vi "Calc Frame Data .vi"(9 "Rotation Center From Robot Center":T6, 11 "Frame":T5={"Length"=5.0, "Width"=1020.0}) -> (3 "Frame Rotation Set Out":T1 {"Back Right"."Angle" scale format="%.3f"; "Back Right"."Velocity" scale=-1.0..1.0 scale format="%.1f"; "Back Left"."Angle" scale format="%.3f"; "Back Left"."Velocity" scale=-1.0..1.0 scale format="%.1f"; "Front Left"."Angle" scale format="%.3f"; "Front Left"."Velocity" scale=-1.0..1.0 scale format="%.1f"; "Front Right"."Angle" scale format="%.3f"; "Front Right"."Velocity" scale=-1.0..1.0 scale format="%.1f"})   [LabVIEW 2023, in "TShirtWork-SwerveDrive_ACT_ts.lvlib"]
uses:
  TShirtWork-SwerveDrive_ACT_ts.lvlib
  Shared Code/TypeDefs/Cluster_X-Y.ctl
  Type Defs/Cluster_Length and Width.ctl
  Shared Code/TypeDefs/Cluster_Swerve 4 Steer and Velocity.ctl
  Shared Code/TypeDefs/Cluster_Module Velocity-Direction-Rotations.ctl
  Shared Code/TypeDefs/Level_Velocity plus-minus 1.ctl
  Shared Code/TypeDefs/Dial_Compase heading unit circle CCW positive.ctl
  Shared Code/TypeDefs/ENUM_Module Position.ctl
  4e8dd0b3-85a2-4953-8cd2-444eefea6a12.vi
  5d84ef4d-5a06-42ca-b3c1-887b7d6f96c4.vi
panel:
  # "\"Front\" of Robot"
  # "Right Hand Rule"
  # "X"
  # "+CCW"
  # "Y"
  # "(0,0)"
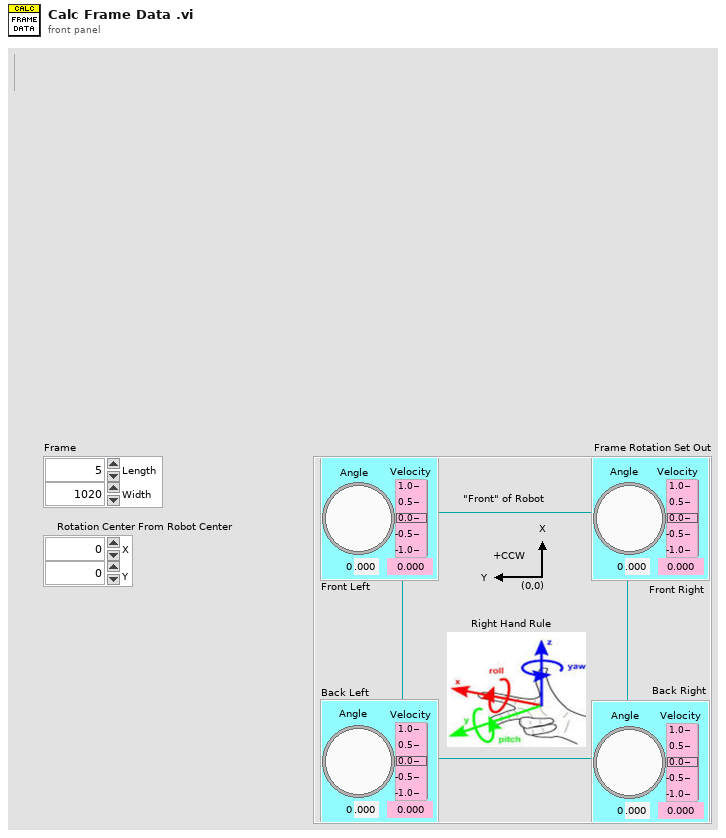
[diagram p1: front panel]
types:
  T1 = typedef "Cluster_Swerve 4 Steer and Velocity.ctl" = cluster{"Front Right":T2, "Front Left":T2, "Back Left":T2, "Back Right":T2}
  T2 = typedef "Cluster_Module Velocity-Direction-Rotations.ctl" = cluster{"Velocity":T3, "Angle":T4, "Rotations Count":dbl}
  T3 = typedef "Level_Velocity plus-minus 1.ctl" = dbl
  T4 = typedef "Dial_Compase heading unit circle CCW positive.ctl" = dbl
  T5 = typedef "Cluster_Length and Width.ctl" = cluster{"Length":dbl, "Width":dbl}
  T6 = typedef "Cluster_X-Y.ctl" = cluster{"X":dbl, "Y":dbl}
  T7 = typedef "ENUM_Module Position.ctl" = enum16{"Left-Front", "Right-Front", "Left-Back", "Right-Back"}
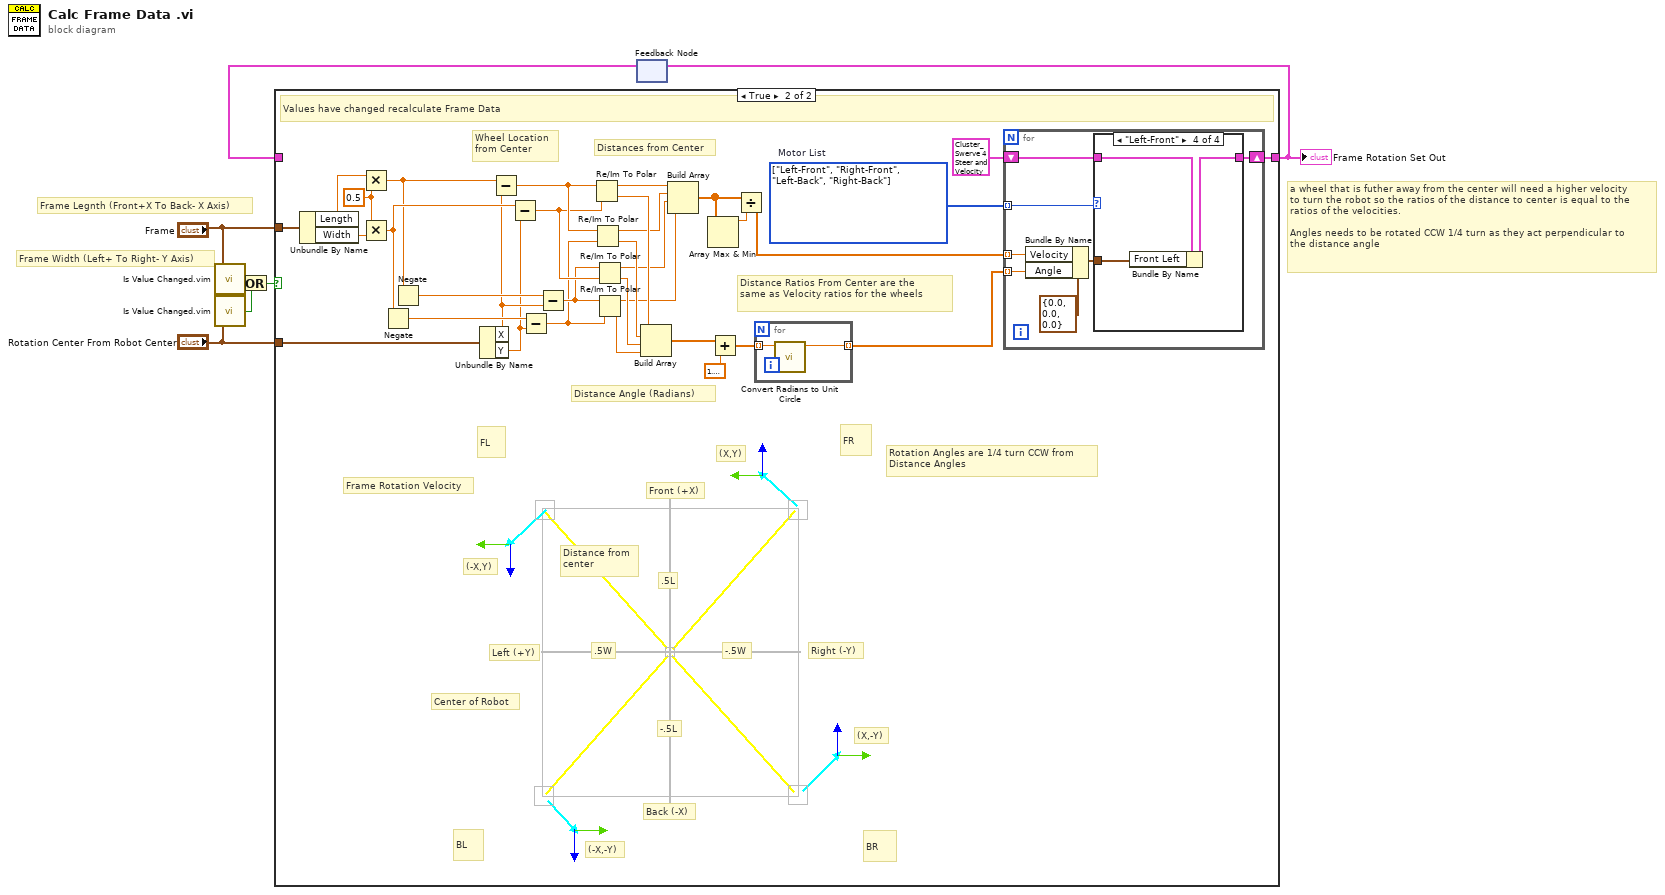
[diagram p0: block diagram]
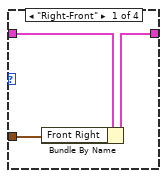
[diagram p3: hidden frame]
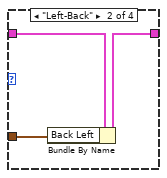
[diagram p4: hidden frame]
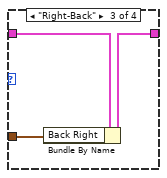
[diagram p5: hidden frame]
diagram:
  # "a wheel that is futher away from the center will need a higher velocity\nto turn the robot so the ratios of the distance to center is equal to the\nratios of the velocities. \n\nAngles needs to be rotated CCW 1/4 turn as they act perpendicular to\nthe distance angle"
  # "Frame Width (Left+ To Right- Y Axis)"
  # "Frame Legnth (Front+X To Back- X Axis)"
  n1 = call "Is Value Changed.vim"("value"="Frame") -> ("changed or first call?"=w7:bool)
  n2 = call "Is Value Changed.vim"("value"="Rotation Center From Robot Center") -> ("changed or first call?"=w2:bool)
  n3 = Or(x=w7, y=w2) -> (x .or. y?=w3:bool)
  n4 = feedback #1() -> (w6:T1)  [unwired: 1 in]
  n5 = case shown="True" w3 {
    tunnel: w6 -> [w8 _]
    tunnel: "Frame" -> [_ w32]
    tunnel: "Rotation Center From Robot Center" -> [_ w29]
    tunnel: [w8 w12] -> w1
    frame False {
      # "Input Values have not changed use previous calculated values"
    }
    frame True {
      w9 = T7[] [enum."Left-Front", enum."Right-Front", enum."Left-Back", enum."Right-Back"] items=["Left-Front", "Right-Front", "Left-Back", "Right-Back"]  # Motor List
      w37 = 0.5 ("y")
      # "Rotation Angles are 1/4 turn CCW from\nDistance Angles"
      # "Center of Robot"
      # "Distance Angle (Radians)"
      # "Distance from\ncenter"
      # "Frame Rotation Velocity"
      # "(X,Y)"
      # "(X,-Y)"
      # "(-X,-Y)"
      # "(-X,Y)"
      # "Right (-Y)"
      # "Left (+Y)"
      # "Back (-X)"
      # "Front (+X)"
      # "BR"
      # "BL"
      # "FL"
      # "FR"
      # ".5W"
      # "-.5W"
      # "-.5L"
      # ".5L"
      # "Distance Ratios From Center are the \nsame as Velocity ratios for the wheels"
      # "Distances from Center"
      # "Wheel Location\nfrom Center"
      # "Values have changed recalculate Frame Data"
      n6 = Unbundle By Name(w32) -> ("Length"=w31:dbl, "Width"=w30:dbl)
      n7 = Multiply(x=w31, y=w37) -> (x*y=w38:dbl)
      n8 = Multiply(x=w37, y=w30) -> (x*y=w39:dbl)
      n9 = Negate(x=w39) -> (-x=w41:dbl)
      n10 = Negate(x=w38) -> (-x=w40:dbl)
      n11 = Unbundle By Name(w29) -> ("X"=w28:dbl, "Y"=w27:dbl)
      n12 = Subtract(x=w38, y=w28) -> (x-y=w26:dbl)
      n13 = Subtract(x=w39, y=w27) -> (x-y=w25:dbl)
      n14 = Subtract(x=w41, y=w27) -> (x-y=w23:dbl)
      n15 = Subtract(x=w40, y=w28) -> (x-y=w24:dbl)
      n16 = Re/Im To Polar(2:w25, 3:w26) -> (0:w21:dbl, 1:w22:dbl)
      n17 = Re/Im To Polar(2:w23, 3:w26) -> (0:w19:dbl, 1:w20:dbl)
      n18 = Re/Im To Polar(2:w25, 3:w24) -> (0:w17:dbl, 1:w18:dbl)
      n19 = Re/Im To Polar(2:w23, 3:w24) -> (0:w15:dbl, 1:w16:dbl)
      n20 = Build Array(w21, w19, w17, w15) -> (w34:dbl[])
      n21 = Build Array(w22, w20, w18, w16) -> (w36:dbl[])
      n22 = Array Max & Min(array=w36) -> (max value=w35:dbl)  [unwired: 3 out]
      n23 = Add(x=w34, y=1.5707963267948966) -> (x+y=w14:dbl[])
      n24 = Divide(x=w36, y=w35) -> (x/y=w10:dbl[])
      n25 = for {
        tunnel: w14 -> [w62] mode=indexing
        tunnel: [w61] -> w11 mode=indexing
        n26 = call "Convert Radians to Unit Circle.vi"("Radians"=w62) -> ("Unit Circle"=w61:dbl)  [unwired: 10 in]
      }
      n27 = for {
        shift-right: [w47] -> w12
        shift-left: T1 {"Front Right"={"Velocity"=0.0, "Angle"=0.0, "Rotations Count"=0.0}, "Front Left"={"Velocity"=0.0, "Angle"=0.0, "Rotations Count"=0.0}, "Back Left"={"Velocity"=0.0, "Angle"=0.0, "Rotations Count"=0.0}, "Back Right"={"Velocity"=0.0, "Angle"=0.0, "Rotations Count"=0.0}} ("Swerve Request Out") -> [w48]
        tunnel: w11 -> [w42] mode=indexing
        tunnel: w10 -> [w43] mode=indexing
        tunnel: w9 -> [w46] mode=indexing
        n28 = Bundle By Name(cluster=T2 {"Velocity"=0.0, "Angle"=0.0, "Rotations Count"=0.0} ("Front Right"), "Velocity"=w43, "Angle"=w42) -> (w44:T2)
        n29 = case shown="\"Left-Front\"" w46 {
          tunnel: w48 -> [w51 w54 w57 w60]
          tunnel: [w50 w53 w56 w59] -> w47
          tunnel: w44 -> [w49 w52 w55 w58]
          frame "Right-Front" {
            n30 = Bundle By Name(cluster=w51, "Front Right"=w49) -> (w50:T1)
          }
          frame "Left-Back" {
            n31 = Bundle By Name(cluster=w54, "Back Left"=w52) -> (w53:T1)
          }
          frame "Right-Back" {
            n32 = Bundle By Name(cluster=w57, "Back Right"=w55) -> (w56:T1)
          }
          frame "Left-Front" {
            n33 = Bundle By Name(cluster=w60, "Front Left"=w58) -> (w59:T1)
          }
        }
      }
    }
  }
  "Frame Rotation Set Out" <- w1
  n34 = feedback-in #1(w1) -> ()
